vi "Count Ways to Win.vi"(9 "previous record":i64, 11 "time":i64) -> (3 "wins":i32)   [LabVIEW 2022 SP3]
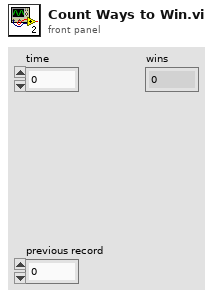
[diagram p1: front panel]
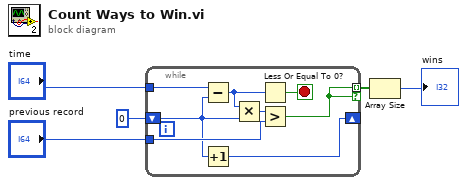
[diagram p0: block diagram]
diagram:
  n1 = while {
    tunnel: "previous record" -> [w12]
    tunnel: "time" -> [w10]
    tunnel: [w11] -> w1 mode=indexing if=w11
    shift-right: [w8] -> _
    shift-left: i64 0 ("default value 1") -> [w9]
    stop <- w6 stop-if-true
    n2 = Subtract(x=w10, y=w9) -> (x-y=w7:i64)
    n3 = Increment(x=w9) -> (x+1=w8:i64)
    n4 = Multiply(x=w7, y=w9) -> (x*y=w13:i64)
    n5 = Less Or Equal To 0?(x=w7) -> (x <= 0?=w6:bool)
    n6 = Greater?(x=w13, y=w12) -> (0:w11:bool)
  }
  n7 = Array Size(array=w1) -> (size(s)=→"wins":i32)
